vi "Flat_Sequence.vi"() -> ()   [LabVIEW 2016]
panel:
  out "x+y":dbl
  out "Triangle":dynamicdata(graph)
  out "Sine":dynamicdata(graph)
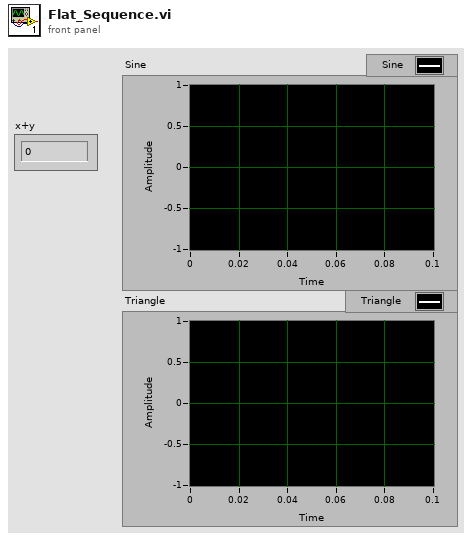
[diagram p1: front panel]
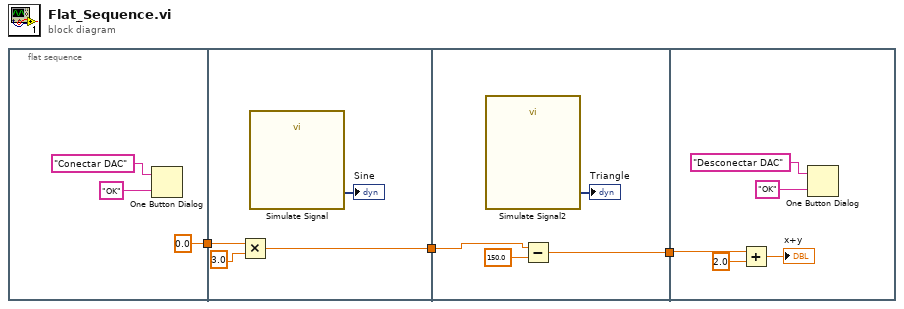
[diagram p0: block diagram]
diagram:
  n1 = flat-sequence {
    tunnel: [0.0] -> w3
    tunnel: w3 -> [w8]
    tunnel: [w7] -> w2
    tunnel: w2 -> [w12]
    tunnel: [w11] -> w1
    tunnel: w1 -> [w17]
    frame #0 {
      n2 = One Button Dialog(message="Conectar DAC", button name ("OK")="OK") -> ()  [unwired: 1 out]
    }
    frame #1 {
      n3 = Multiply(x=w8, y=3.0) -> (x*y=w7:dbl)
      n4 = call "Simulate Signal"() -> ("Sine"=→"Sine":dynamicdata)  [unwired: 14 in, 1 out]
    }
    frame #2 {
      n5 = call "Simulate Signal2"() -> ("Triangle"=→"Triangle":dynamicdata)  [unwired: 14 in, 1 out]
      n6 = Subtract(x=w12, y=150.0) -> (x-y=w11:dbl)
    }
    frame #3 {
      n7 = Add(x=w17, y=2.0) -> (x+y=→"x+y":dbl)
      n8 = One Button Dialog(message="Desconectar DAC", button name ("OK")="OK") -> ()  [unwired: 1 out]
    }
  }
